vi "LvMPDC_CMD_stop.vi"(6 "timeout_ms":i32=25000, 8 "error in (no error)":errorcluster, 9 "ReadBytes":i32=1024, 11 "Connect ID":refnum<k5>) -> (0 "error out":errorcluster, 3 "Connect ID out":refnum<k5>)   [LabVIEW 2012]
panel:
  # "LvMPDC:: CMD stop"
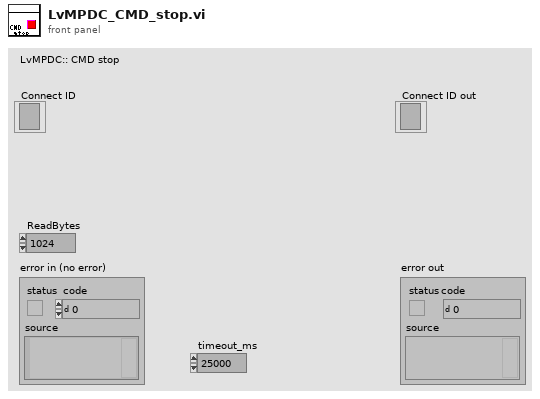
[diagram p1: front panel]
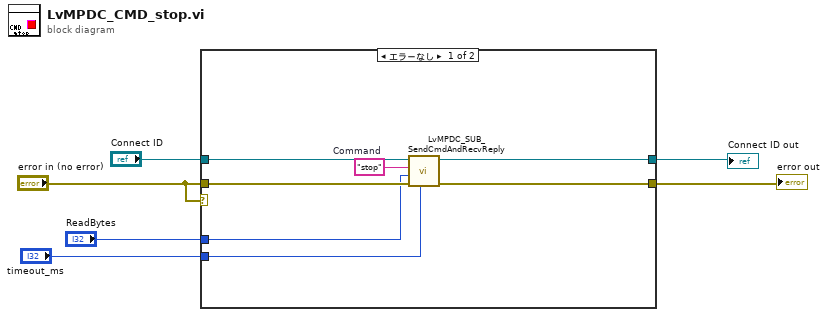
[diagram p0: block diagram]
diagram:
  n1 = case shown="エラーなし" "error in (no error)" {
    tunnel: "Connect ID" -> [w11 w15]
    tunnel: "error in (no error)" -> [w13 w14]
    tunnel: [w10 w15] -> w5
    tunnel: [w12 w14] -> w4
    tunnel: "timeout_ms" -> [w7 _]
    tunnel: "ReadBytes" -> [w8 _]
    frame No Error {
      w9 = "stop"  # Command
      n2 = call "LvMPDC_SUB_SendCmdAndRecvReply.vi"("timeout_ms"=w7, "error in (no error)"=w13, "ReadBytes"=w8, "Command"=w9, "Connect ID"=w11) -> ("error out"=w12:errorcluster, "Connect ID out"=w10:refnum<k5>)  [unwired: 4 in, 1 out]
    }
    frame Error {
    }
  }
  "Connect ID out" <- w5
  "error out" <- w4
